vi "Get Channel Reading.vi"(8 "error in":errorcluster, 10 "Channel":string, 11 "Buffer Lossless Bin in":refnum<class "Buffer Lossless Digital.lvclass">) -> (0 "error out":errorcluster, 1 "empty?":bool, 2 "Reading":digitalwaveform(waveform), 3 "Buffer Lossless Bin out":refnum<class "Buffer Lossless Digital.lvclass">)   [LabVIEW 2024, in "Buffer Lossless Digital.lvclass"]
uses:
  Buffer Lossless Digital.lvclass
  Buffer Lossless Digital.lvclass/Buffer Lossless Digital.ctl
  <vilib>/Waveform/DWDTOps.llb/DWDT Append Digital Samples.vi
  <vilib>/Waveform/DWDTOps.llb/DWDT Digital Size.vi
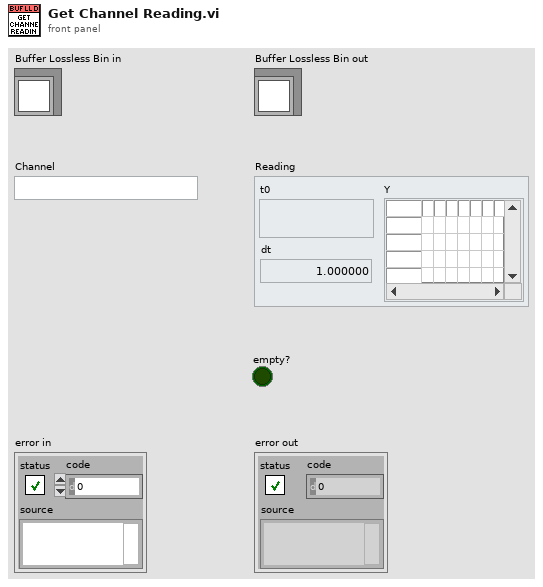
[diagram p1: front panel]
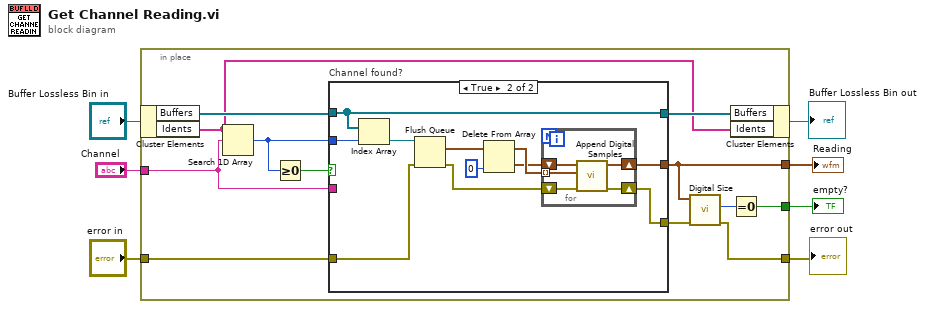
[diagram p0: block diagram]
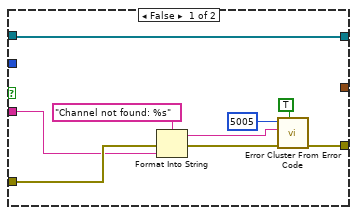
[diagram p2: hidden frame]
diagram:
  n1 = in-place {
    in-place-border: "error in" -> [w13]
    in-place-border: [w8] -> w2
    in-place-border: "Channel" -> [w14]
    in-place-border: [w12] -> w4
    in-place-border: [w10] -> w1
    n2 = in-place-cluster #1("Buffer Lossless Bin in") -> ("Buffers"=w17:refnum<queue>[], "Idents"=w15:string[])
    n3 = Search 1D Array(1D array=w15, element=w14) -> (index of element=w19:i32)  [unwired: 1 in]
    n4 = Greater Or Equal To 0?(x=w19) -> (x >= 0?=w18:bool)
    n5 = case "Channel found?" shown="True" w18 {
      tunnel: w13 -> [w23 w39]
      tunnel: [w22 w38] -> w9
      tunnel: w17 -> [w21 w29]
      tunnel: w19 -> [_ w35]
      tunnel: [w21 w29] -> w16
      tunnel: [_ w37] -> w12
      tunnel: w14 -> [w20 _]
      frame False {
        n6 = Format Into String(format string="Channel not found: %s", error in=w23, w20) -> (resulting string=w24:string, error out=w26:errorcluster)  [unwired: 1 in]
        n7 = call <vilib>:"Error Cluster From Error Code.vi"("show call chain? (False)"=TRUE, "error in (no error)"=w26, "error message (\"\")"=w24, "error code (0)"=5005) -> ("error out"=w22:errorcluster)  [unwired: 5 in]
      }
      frame True {
        n8 = Index Array(array=w29, index=w35) -> (element=w36:refnum<queue>)
        n9 = Flush Queue(queue=w36, error in (no error)=w39) -> (remaining elements=w33:digitalwaveform[], error out=w34:errorcluster)  [unwired: 1 out]
        n10 = Delete From Array(array=w33, index=0) -> (deleted portion=w30:digitalwaveform, array with subset deleted=w31:digitalwaveform[])  [unwired: 1 in]
        n11 = for {
          tunnel: w31 -> [w41] mode=indexing
          shift-right: [w42] -> w37
          shift-left: w30 -> [w40]
          shift-right: [w43] -> w38
          shift-left: w34 -> [w44]
          n12 = call-poly <vilib>:"Append Digital Samples.vi"("error in (no error)"=w44, "digital waveform B"=w41, "digital waveform A"=w40) -> ("error out"=w43:errorcluster, "digital waveform out"=w42:digitalwaveform)  [unwired: 7 in]
        }
      }
    }
    n13 = call-poly <vilib>:"Digital Size.vi"("error in (no error)"=w9, "digital waveform in"=w12) -> ("error out"=w8:errorcluster, "number of samples"=w11:i32)  [unwired: 6 in, 2 out]
    n14 = in-place-cluster #1("Buffers"=w16, "Idents"=w15) -> (→"Buffer Lossless Bin out":refnum<class "Buffer Lossless Digital.lvclass">)
    n15 = Equal To 0?(x=w11) -> (x = 0?=w10:bool)
  }
  "error out" <- w2
  "Reading" <- w4
  "empty?" <- w1
